vi "Read Is OK.vi"(8 "Error In":errorcluster, 11 "Reader In":refnum<class "Reader.lvclass">) -> (0 "Error Out":errorcluster, 2 "OK":bool, 3 "Reader Out":refnum<class "Reader.lvclass">)   [LabVIEW 2019, in "LabPack.lvlib" / "Reader.lvclass"]
doc: "Checks if the internal decoder is OK."
uses:
  Reader.lvclass
  Reader.lvclass/Reader.ctl
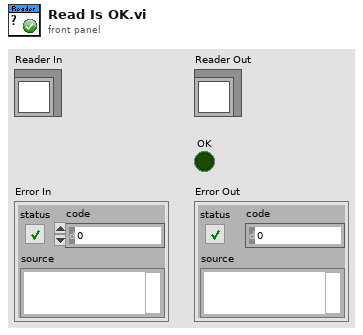
[diagram p1: front panel]
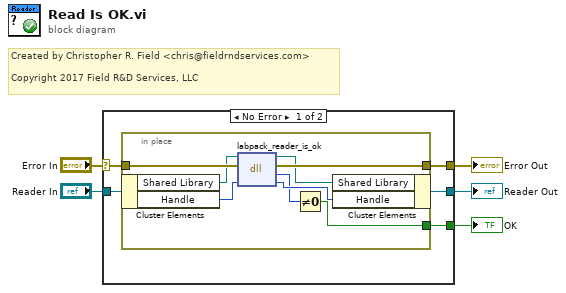
[diagram p0: block diagram]
diagram:
  # "Created by Christopher R. Field <chris@fieldrndservices.com>\n\nCopyright 2017 Field R&D Services, LLC"
  n1 = case shown="No Error" "Error In" {
    selector: "Error In" -> [w10 w20]
    tunnel: "Reader In" -> [w7 w19]
    tunnel: [w9 w20] -> w4
    tunnel: [w8 _] -> w3
    tunnel: [w6 w19] -> w1
    frame No Error {
      n2 = in-place {
        in-place-border: w10 -> [w18]
        in-place-border: [w17] -> w9
        in-place-border: [w13] -> w8
        n3 = in-place-cluster #1(w7) -> ("Shared Library"=w12:path, "Handle"=w11:u64)
        n4 = dll-call lib="D:/Users/cfield/Code/MessagePack/LabPack/LabVIEW/trunk/src/LabPack/Private/labpack-x64.dll" fn="labpack_reader_is_ok"(path in=w12, error in=w18, "reader"=w11) -> (path out=w15:path, error out=w17:errorcluster, "return type"=w14:i32, "reader"=w16:u64)  [unwired: 1 in]
        n5 = Not Equal To 0?(x=w14) -> (x != 0?=w13:bool)
        n6 = in-place-cluster #1("Shared Library"=w15, "Handle"=w16) -> (w6:refnum<class "Reader.lvclass">)
      }
    }
    frame Error {
    }
  }
  "Error Out" <- w4
  "OK" <- w3
  "Reader Out" <- w1
